vi "dfd_Utility I32 x I32 (MSBs).vi"(1 "y[I32]":i32, 2 "x[I32]":i32) -> (0 "x*y[I32 MSB]":i32)   [LabVIEW 2017, in "NI_DigFilterLicensed.lvlib"]
uses:
  <vilib>/addons/Digital Filter Design/NI_DigFilterLicensed.lvlib
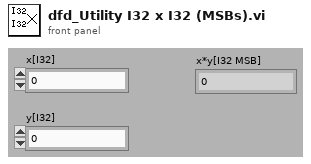
[diagram p1: front panel]
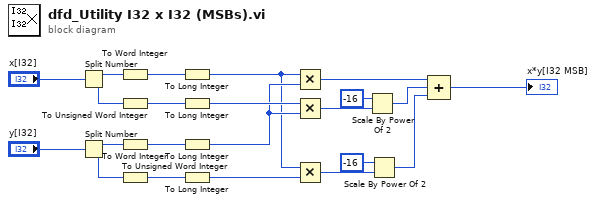
[diagram p0: block diagram]
diagram:
  n1 = Split Number(x="x[I32]") -> (hi(x)=w22:u16, lo(x)=w18:u16)
  n2 = Split Number(x="y[I32]") -> (hi(x)=w21:u16, lo(x)=w17:u16)
  n3 = To Word Integer(number=w22) -> (16bit integer=w16:i16)
  n4 = To Unsigned Word Integer(number=w18) -> (unsigned 16bit integer=w14:u16)
  n5 = To Word Integer(number=w21) -> (16bit integer=w15:i16)
  n6 = To Unsigned Word Integer(number=w17) -> (unsigned 16bit integer=w13:u16)
  n7 = To Long Integer(number=w16) -> (32bit integer=w9:i32)
  n8 = To Long Integer(number=w14) -> (32bit integer=w12:i32)
  n9 = To Long Integer(number=w15) -> (32bit integer=w11:i32)
  n10 = To Long Integer(number=w13) -> (32bit integer=w10:i32)
  n11 = Multiply(x=w9, y=w11) -> (x*y=w8:i32)
  n12 = Multiply(x=w12, y=w11) -> (x*y=w7:i32)
  n13 = Multiply(x=w9, y=w10) -> (x*y=w5:i32)
  n14 = Scale By Power Of 2(n=-16, x=w7) -> (x*2^n=w3:i32)
  n15 = Scale By Power Of 2(n=-16, x=w5) -> (x*2^n=w2:i32)
  n16 = Compound Arithmetic op=ADD(w8, w3, w2) -> (→"x*y[I32 MSB]":i32)
